vi "Mirror Image(1 bit Horizontal).vi"(8 "错误输入":errorcluster, 11 "image In":T1 caption="Image in") -> (0 "错误输出":errorcluster, 3 "image out":T1 caption="Image out")   [LabVIEW 2011]
uses:
  <vilib>/picture/picture.llb/imagedata.ctl
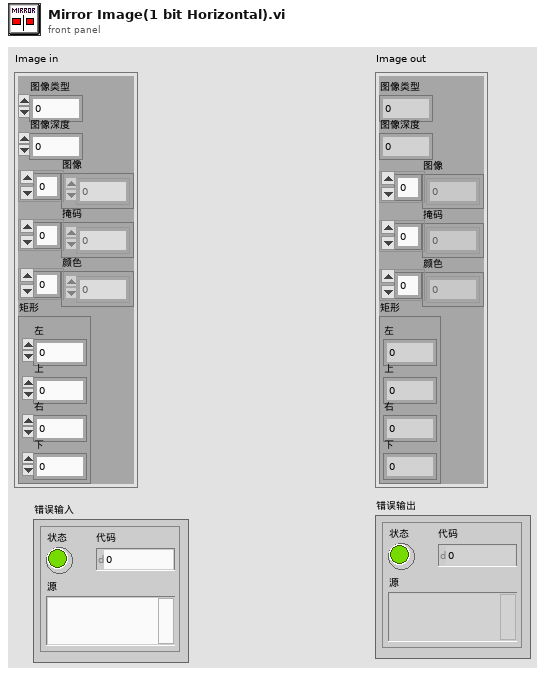
[diagram p1: front panel]
types:
  T1 = typedef "imagedata.ctl" = cluster{"image type":i32, "image depth":i32, "image":u8[], "mask":u8[], "colors":u32[], "Rectangle":cluster{"left":i16, "top":i16, "right":i16, "bottom":i16}}
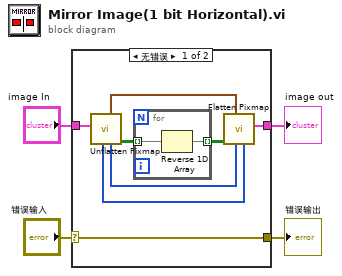
[diagram p0: block diagram]
diagram:
  n1 = case shown="无错误" "错误输入" {
    selector: "错误输入" -> [w9 w15]
    tunnel: [w9 w15] -> w3
    tunnel: "image In" -> [w8 _]
    tunnel: [w7 _] -> w1
    frame No Error {
      n2 = call <vilib>:"Unflatten Pixmap.vi"("image data"=w8) -> ("1-bit pixmap"=w6:bool[][], "colors"=w12:u32[], "top left"=w10:cluster{"x":i16, "y":i16}, "mask"=w11:u8[])  [unwired: 4 in, 3 out]
      n3 = for {
        tunnel: w6 -> [w14] mode=indexing
        tunnel: [w13] -> w5 mode=indexing
        n4 = Reverse 1D Array(array=w14) -> (reversed array=w13:bool[])
      }
      n5 = call <vilib>:"Flatten Pixmap.vi"("mask"=w11, "colors"=w12, "top left"=w10, "1-bit pixmap"=w5) -> ("image data"=w7:T1)  [unwired: 7 in]
    }
    frame Error {
    }
  }
  "错误输出" <- w3
  "image out" <- w1
